vi "Fetch Histogram.vi"(8 "error in (no error)":errorcluster {"code" format="%.0x"}, 9 "Bin Range (0: 8A)":i32(ring) items=["8 A", "0.0039 A"], 10 "Channel Name (1)":string="1", 11 "VISA resource name":refnum<visa-resource-name>) -> (0 "error out":errorcluster {"code" format="%.0x"}, 2 "Bin Data":dbl[](array[numeric]) format="%^.3e", 3 "VISA resource name out":refnum<visa-resource-name>)   [LabVIEW 2016, in "Agilent N6700 Series.lvlib"]
doc: "Returns the bin data from the current histogram.\n\n<b>Notes:</b>\n(1) This VI only applies to models N678xA SMU that have the Data Logger function installed.\n(2) This VI only applies to the N6705B and N6705C DC Power Analyzer."
uses:
  <instrlib>/Agilent N6700 Series/Agilent N6700 Series.lvlib
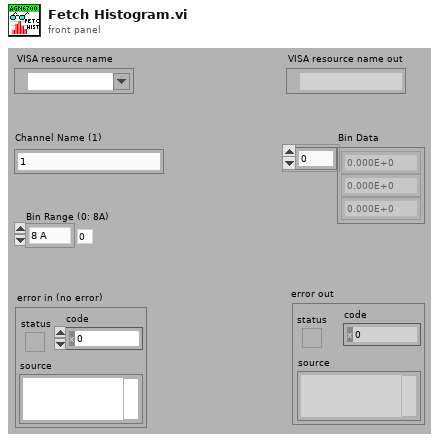
[diagram p1: front panel]
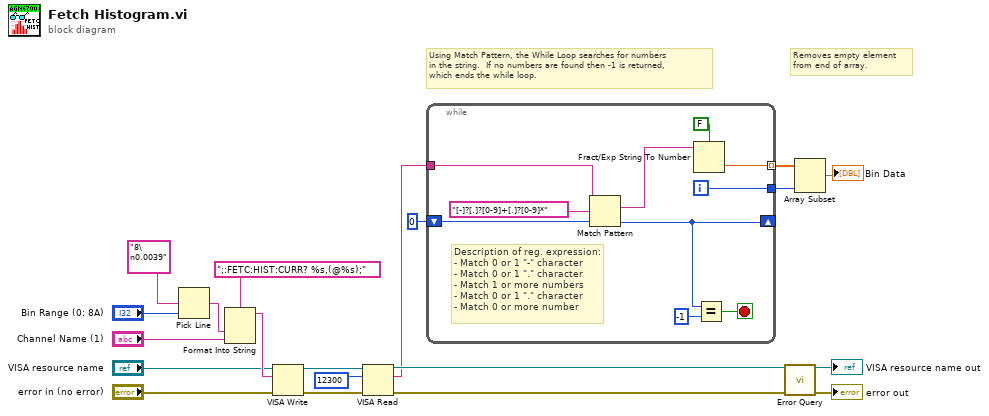
[diagram p0: block diagram]
diagram:
  # "Removes empty element\nfrom end of array."
  # "Using Match Pattern, the While Loop searches for numbers\nin the string.  If no numbers are found then -1 is returned,\nwhich ends the while loop."
  n1 = Pick Line(multi-line string="8\n0.0039", line index="Bin Range (0: 8A)") -> (output string=w8:string)  [unwired: 1 in]
  n2 = Format Into String(format string=";:FETC:HIST:CURR? %s,(@%s);", w8, "Channel Name (1)") -> (resulting string=w16:string)  [unwired: 2 in, 1 out]
  n3 = VISA Write(VISA resource name="VISA resource name", write buffer=w16, error in (no error)="error in (no error)") -> (VISA resource name out=w19:refnum<visa-resource-name>, error out=w18:errorcluster)  [unwired: 1 out]
  n4 = VISA Read(VISA resource name=w19, byte count=u32 12300, error in (no error)=w18) -> (VISA resource name out=w11:refnum<visa-resource-name>, read buffer=w2:string, error out=w10:errorcluster)  [unwired: 1 out]
  n5 = while {
    tunnel: [w30] -> w4
    shift-left: 0 -> [w25]
    shift-right: [w24] -> _
    tunnel: [w28] -> w5 mode=indexing
    tunnel: w2 -> [w22]
    i -> [w30]
    stop <- w27 stop-if-true
    # "Description of reg. expression:\n- Match 0 or 1 \"-\" character\n- Match 0 or 1 \".\" character\n- Match 1 or more numbers\n- Match 0 or 1 \".\" character\n- Match 0 or more number"
    n6 = Match Pattern(string=w22, regular expression="[-]?[.]?[0-9]+[.]?[0-9]*", offset (0)=w25) -> (match substring=w23:string, offset past match=w24:i32)  [unwired: 2 out]
    n7 = Fract/Exp String To Number(use system decimal point (T)=FALSE, string=w23) -> (number=w28:dbl)  [unwired: 2 in, 1 out]
    n8 = Equal?(x=w24, y=-1) -> (x = y?=w27:bool)
  }
  n9 = call <instrlib>:"Error Query.vi"("VISA resource name"=w11, "error in (no error)"=w10) -> ("VISA resource name out"=→"VISA resource name out":refnum<visa-resource-name>, "error out"=→"error out":errorcluster)  [unwired: 10 in, 2 out]
  n10 = Array Subset(array=w5, length=w4) -> (→"Bin Data":dbl[])  [unwired: 1 in]
